vi "Initialize.vi"(8 "Phi":dbl, 9 "T":dbl, 10 "A":dbl) -> (3 "Sine out":refnum<class "Sine.lvclass">)   [LabVIEW 2020, in "Sine.lvclass"]
uses:
  Sine.lvclass
  Sine.lvclass/Sine.ctl
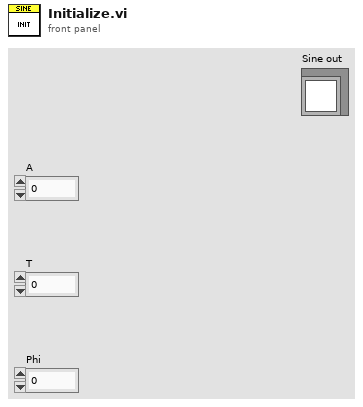
[diagram p1: front panel]
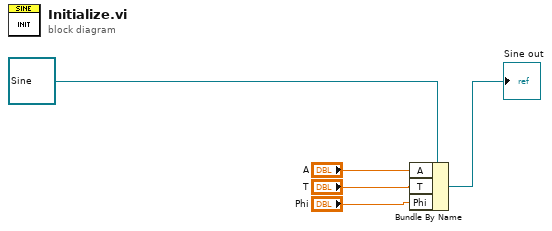
[diagram p0: block diagram]
diagram:
  n1 = Bundle By Name(cluster=refnum<class "Sine.lvclass"> refnum ("Sine in"), "A"="A", "T"="T", "Phi"="Phi") -> (→"Sine out":refnum<class "Sine.lvclass">)
